vi "Enqueue High Priority.vi"(8 "Error In":errorcluster, 10 "Data":variant, 11 "Command":T1) -> (0 "Error Out":errorcluster)   [LabVIEW 2016, in "Anti-Spam Tester (AST).lvlib" / "AST MHL Queue.lvclass"]
doc: "Issues a command by enqueuing into the module's command queue. The command should be received by calling the 'Dequeue' VI.\n\nUses 'Enqueue Element At Opposite End' to enqueue a high priority message.\n\nRecommendation: Use the regular 'Enqueue' VI for most messages. Use the 'Enqueue High Priority' for a selected few messages, usually messages such as 'Abort' or 'Exit App'."
uses:
  AST MHL Queue.lvclass
  Message (cluster).ctl
  Command (enum).ctl
  Queue Reference (library variable).vi
panel:
  # "Input\nInputs to the VI"
  # "Development\nControls or indicators that are useful for development or testing, but which are not outputs of the VI."
  # "Output\nOutputs of the VI"
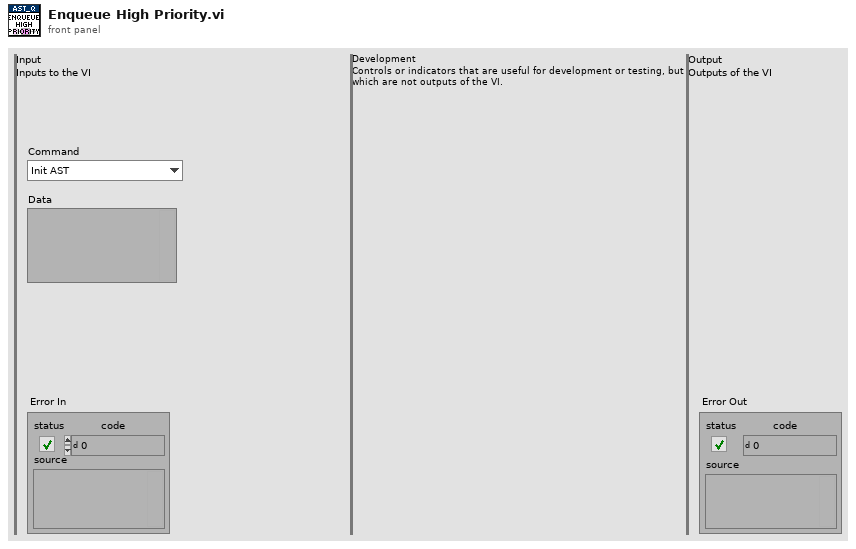
[diagram p1: front panel]
types:
  T1 = typedef "Anti-Spam Tester (AST).lvlib/AST MHL Queue.lvclass/Command (enum).ctl" = enum16{"Init AST", "Close AST", "Config GUI - Init", "Config GUI - Spamming Has Started", "Config GUI - Spamming Has Stopped", "Spam"}
  T2 = typedef "Anti-Spam Tester (AST).lvlib/AST MHL Queue.lvclass/Message (cluster).ctl" = cluster{"Command":T1, "Data":variant}
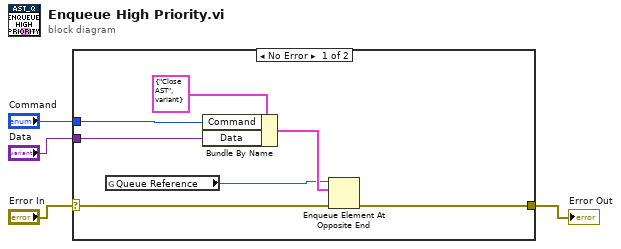
[diagram p0: block diagram]
diagram:
  n1 = case shown="No Error" "Error In" {
    selector: "Error In" -> [w11 w12]
    tunnel: [w10 w12] -> w3
    tunnel: "Command" -> [w7 _]
    tunnel: "Data" -> [w6 _]
    frame No Error {
      n2 = global read "Queue Reference (library variable).vi" "Queue Reference"() -> (w5:refnum<queue>)
      n3 = Bundle By Name(cluster=T2 {"Command"=enum."Close AST", "Data"=variant} ("Queue Message"), "Command"=w7, "Data"=w6) -> (w8:T2)
      n4 = Enqueue Element At Opposite End(queue=w5, element=w8, error in (no error)=w11) -> (error out=w10:errorcluster)  [unwired: 1 in, 2 out]
    }
    frame Error {
    }
  }
  "Error Out" <- w3
